vi "Mono_Query.vi"(8 "error in (no error) 2":errorcluster, 11 "CmdLib In":refnum<k24>) -> (0 "error out 2":errorcluster, 3 "CmdLib Out":refnum<k24>)   [LabVIEW 2023]
uses:
  E:/Old PC/desktop/Sensitive EQE Stuff/S-EQE (YJ)/Mono vi (YJ)/Cornerstone.dll
panel:
  out "getQuery":string
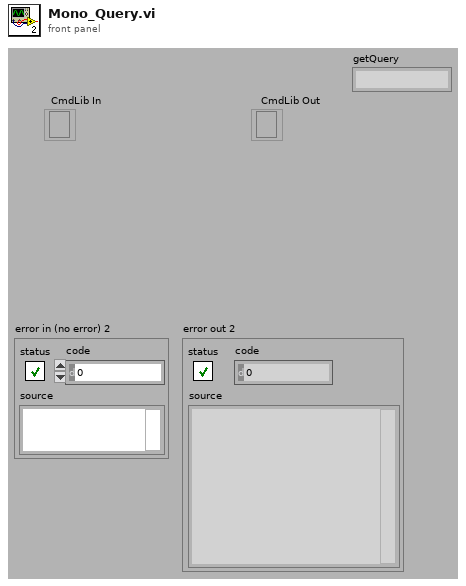
[diagram p1: front panel]
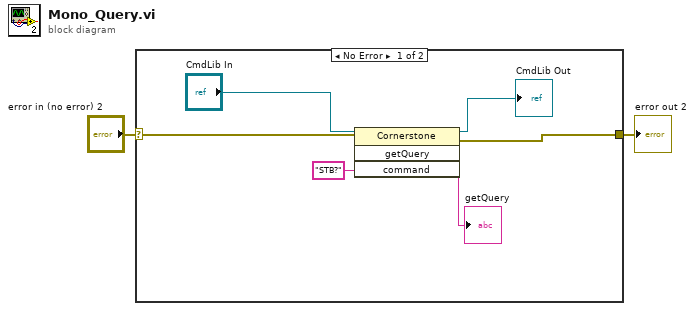
[diagram p0: block diagram]
diagram:
  n1 = case shown="No Error" "error in (no error) 2" {
    selector: "error in (no error) 2" -> [w8 w9]
    tunnel: [w5 w9] -> w1
    frame No Error {
      n2 = invoke class="Cornerstone" method="getQuery"(reference="CmdLib In", error in=w8, "command"="STB?") -> (reference out=→"CmdLib Out":refnum<k24>, error out=w5:errorcluster, "getQuery"=→"getQuery":string)  [unwired: 1 in, 1 out]
    }
    frame Error {
    }
  }
  "error out 2" <- w1
